vi "Set A.vi"(8 "error in (no error)":errorcluster, 10 "Numeric":dbl, 11 "ByRef Base in":refnum<class "ByRef Base.lvclass">) -> (0 "error out":errorcluster, 3 "ByRef Base out":refnum<class "ByRef Base.lvclass">)   [LabVIEW 2020, in "ByRef Base.lvclass"]
uses:
  ByRef Base.lvclass
  ByRef Base.lvclass/ByRef Base.ctl
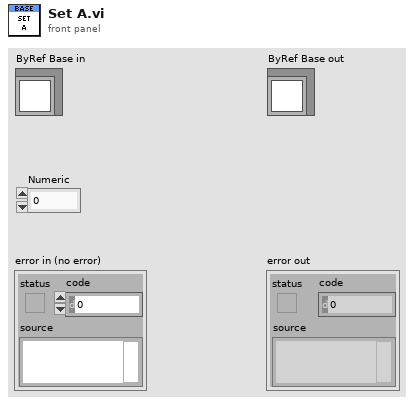
[diagram p1: front panel]
types:
  T1 = typedef "ByRef Base.lvclass/Ref Data.ctl" = cluster{"A":dbl, "B":dbl}
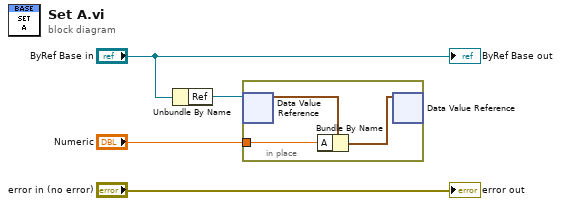
[diagram p0: block diagram]
diagram:
  n1 = Unbundle By Name("ByRef Base in") -> ("Ref"=w3:refnum<data-value>)
  n2 = in-place {
    in-place-border: "Numeric" -> [w5]
    n3 = in-place-dvr #1(w3) -> (w7:T1)  [unwired: 1 out]
    n4 = Bundle By Name(cluster=w7, "A"=w5) -> (w6:T1)
    n5 = in-place-dvr #1(w6) -> ()  [unwired: 2 out]
  }
  "error out" <- "error in (no error)"
  "ByRef Base out" <- "ByRef Base in"
